vi "setpositionabsolute.vi"(8 "error in (no error)":errorcluster, 10 "Position Aboslute":i32, 11 "VISA in":refnum<visa-resource-name>) -> (0 "error out":errorcluster, 3 "VISA out":refnum<visa-resource-name>)   [LabVIEW 2019]
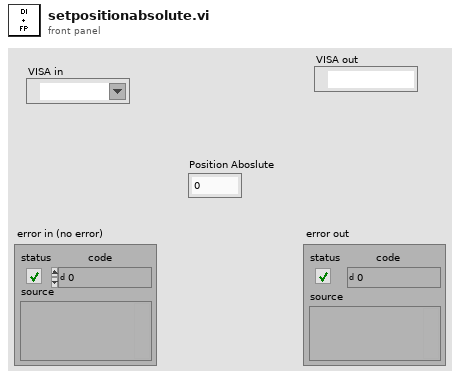
[diagram p1: front panel]
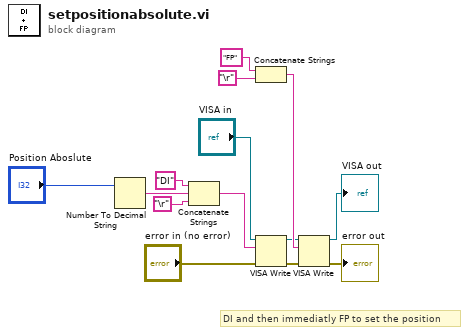
[diagram p0: block diagram]
diagram:
  # "DI and then immediatly FP to set the position"
  n1 = Number To Decimal String(number="Position Aboslute") -> (decimal integer string=w8:string)  [unwired: 1 in]
  n2 = Concatenate Strings("DI", w8, "\r") -> (w14:string)
  n3 = Concatenate Strings("FP", "\r") -> (w5:string)
  n4 = VISA Write(VISA resource name="VISA in", write buffer=w14, error in (no error)="error in (no error)") -> (VISA resource name out=w4:refnum<visa-resource-name>, error out=w3:errorcluster)  [unwired: 1 out]
  n5 = VISA Write(VISA resource name=w4, write buffer=w5, error in (no error)=w3) -> (VISA resource name out=→"VISA out":refnum<visa-resource-name>, error out=→"error out":errorcluster)  [unwired: 1 out]
